vi "FlattenFrame.vi"(2 "Client Frame":T1) -> (16 "flattened frame":string)   [LabVIEW 2017, in "LabVIEW STOMP.lvlib" / "STOMP.lvclass"]
uses:
  STOMP.lvclass
  Typedefs/Type_ClientFrame.ctl
  Typedefs/Type_ClientFrameType.ctl
  Typedefs/Type_FrameHeader.ctl
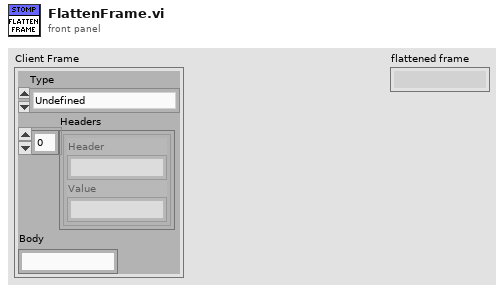
[diagram p1: front panel]
types:
  T1 = typedef "LabVIEW STOMP.lvlib/STOMP.lvclass/Type_ClientFrame.ctl" = cluster{"Type":T2, "Headers":T3[], "Body":string}
  T2 = typedef "LabVIEW STOMP.lvlib/STOMP.lvclass/Type_ClientFrameType.ctl" = enum16{"Undefined", "SEND", "SUBSCRIBE", "UNSUBSCRIBE", "BEGIN", "COMMIT", "ABORT", "ACK", "NACK", "DISCONNECT"}
  T3 = typedef "LabVIEW STOMP.lvlib/STOMP.lvclass/Type_FrameHeader.ctl" = cluster{"Header":string, "Value":string}
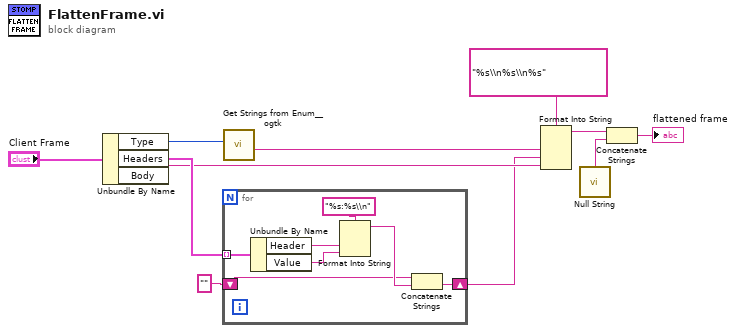
[diagram p0: block diagram]
diagram:
  n1 = Unbundle By Name("Client Frame") -> ("Type"=w11:T2, "Headers"=w8:T3[], "Body"=w7:string)
  n2 = for {
    tunnel: w8 -> [w18] mode=indexing
    shift-right: [w13] -> w1
    shift-left: "" -> [w12]
    n3 = Unbundle By Name(w18) -> ("Header"=w16:string, "Value"=w15:string)
    n4 = Format Into String(format string="%s:%s\\n", w16, w15) -> (resulting string=w14:string)  [unwired: 2 in, 1 out]
    n5 = Concatenate Strings(w12, w14) -> (w13:string)
  }
  n6 = call <userlib>:"Get Strings from Enum__ogtk.vi"("Enum"=w11) -> ("String Value"=w9:string)  [unwired: 7 in, 3 out]
  n7 = Format Into String(format string="%s\\n%s\\n%s", w9, w1, w7) -> (resulting string=w5:string)  [unwired: 2 in, 1 out]
  n8 = call "Null String.vi"() -> ("NULL"=w3:string)  [unwired: 19 in]
  n9 = Concatenate Strings(w5, w3) -> (→"flattened frame":string)
